vi "6.vi"() -> ()   [LabVIEW 2017]
panel:
  out "平均值":dbl
  out "最小值":dbl
  out "最大值":dbl
  out "波形图":dbl[][](graph)
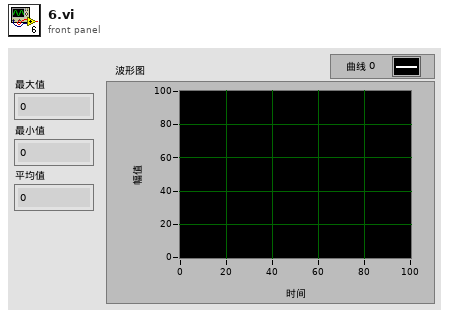
[diagram p1: front panel]
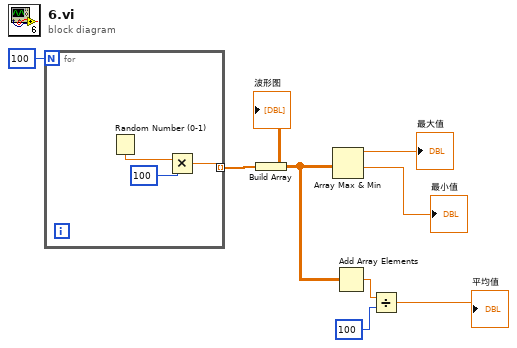
[diagram p0: block diagram]
diagram:
  n1 = for {
    N: 100 -> [_]
    tunnel: [w10] -> w7 mode=indexing
    n2 = Random Number (0-1)() -> (number: 0 to 1=w9:dbl)
    n3 = Multiply(x=w9, y=100) -> (x*y=w10:dbl)
  }
  n4 = Build Array(w7) -> (w1:dbl[][])
  "波形图" <- w1
  n5 = Array Max & Min(array=w1) -> (max value=→"最大值":dbl, min value=→"最小值":dbl)  [unwired: 2 out]
  n6 = Add Array Elements(numeric array=w1) -> (sum=w4:dbl)
  n7 = Divide(x=w4, y=100) -> (x/y=→"平均值":dbl)
